vi "PythonCode.vi"(11 "PythonWrapper in":refnum<class "PythonWrapper.lvclass">) -> (2 "PythonCode":string, 3 "PythonWrapper out":refnum<class "PythonWrapper.lvclass">)   [LabVIEW 2022 SP3, in "PythonWrapper.lvlib" / "PythonWrapper.lvclass"]
uses:
  PythonWrapper.lvclass
  PythonWrapper.lvclass/PythonWrapper.ctl
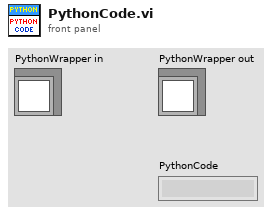
[diagram p1: front panel]
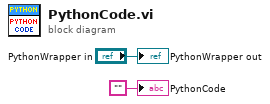
[diagram p0: block diagram]
diagram:
  "PythonWrapper out" <- "PythonWrapper in"
  "PythonCode" <- ""
